vi "example_custom_error.vi"() -> ()   [LabVIEW 2015]
panel:
  out "Error out":errorcluster
  in  "Error in":errorcluster caption="Error in (no error)"
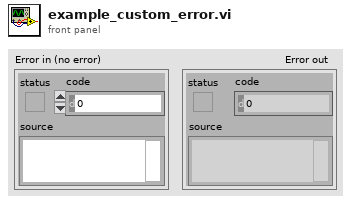
[diagram p1: front panel]
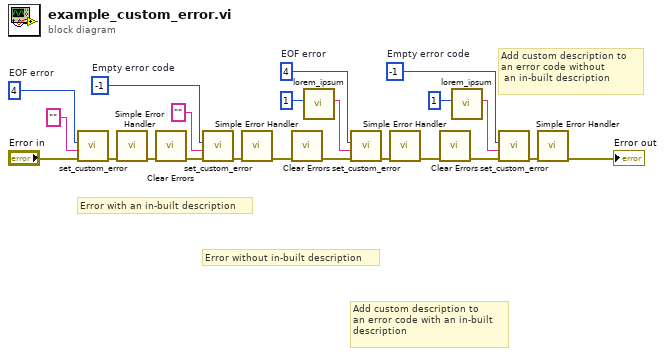
[diagram p0: block diagram]
diagram:
  w7 = -1  # Empty error code
  w8 = 4  # EOF error
  w12 = -1  # Empty error code
  w11 = 4  # EOF error
  # "Add custom description to\nan error code without\n an in-built description"
  # "Add custom description to\nan error code with an in-built\ndescription"
  # "Error without in-built description"
  # "Error with an in-built description"
  n1 = call "set_custom_error.vi"("error in (no error)"="Error in", "custom error description"="" ("Additional info"), "custom code (-1)"=w11) -> ("error out"=w21:errorcluster)  [unwired: 8 in]
  n2 = call <vilib>:"Simple Error Handler.vi"("error in (no error)"=w21) -> ("error out"=w20:errorcluster)  [unwired: 4 in, 4 out]
  n3 = call <vilib>:"Clear Errors.vi"("error in (no error)"=w20) -> ("error out"=w18:errorcluster)  [unwired: 5 in, 1 out]
  n4 = call "set_custom_error.vi"("error in (no error)"=w18, "custom error description"="" ("Additional info"), "custom code (-1)"=w12) -> ("error out"=w19:errorcluster)  [unwired: 8 in]
  n5 = call <vilib>:"Simple Error Handler.vi"("error in (no error)"=w19) -> ("error out"=w17:errorcluster)  [unwired: 4 in, 4 out]
  n6 = call <vilib>:"Clear Errors.vi"("error in (no error)"=w17) -> ("error out"=w15:errorcluster)  [unwired: 5 in, 1 out]
  n7 = call "lorem_ipsum.vi"("N"=1) -> ("lorem ipsum"=w4:string)  [unwired: 10 in]
  n8 = call "set_custom_error.vi"("error in (no error)"=w15, "custom error description"=w4, "custom code (-1)"=w8) -> ("error out"=w16:errorcluster)  [unwired: 8 in]
  n9 = call <vilib>:"Simple Error Handler.vi"("error in (no error)"=w16) -> ("error out"=w14:errorcluster)  [unwired: 4 in, 4 out]
  n10 = call <vilib>:"Clear Errors.vi"("error in (no error)"=w14) -> ("error out"=w10:errorcluster)  [unwired: 5 in, 1 out]
  n11 = call "lorem_ipsum.vi"("N"=1) -> ("lorem ipsum"=w1:string)  [unwired: 10 in]
  n12 = call "set_custom_error.vi"("error in (no error)"=w10, "custom error description"=w1, "custom code (-1)"=w7) -> ("error out"=w13:errorcluster)  [unwired: 8 in]
  n13 = call <vilib>:"Simple Error Handler.vi"("error in (no error)"=w13) -> ("error out"=→"Error out":errorcluster)  [unwired: 4 in, 4 out]
